vi "from string.vi"(8 "error in":errorcluster, 9 "data":string, 10 "version":string, 11 "Fgen configuration":refnum<class "Fgen configuration.lvclass">) -> (0 "error out":errorcluster, 3 "Fgen configuration out":refnum<class "Fgen configuration.lvclass">)   [LabVIEW 2025, in "Fgen.lvlib" / "Fgen configuration.lvclass"]
doc: "Provides an interface for loading a module configuration from a file or other serialized data source. It is recommended that all children of this class store data in two sets--data required for its own initialization, and any data required for parent initialization--and that each implementation uses the <b>Call Parent Method</b> primitive to de-serialize parent information.Copyright 2017 National Instruments Corporation\n\nLicensed under the Apache License, Version 2.0 (the \"License\"); you may not use this file except in compliance with the License. You may obtain a copy of the License at http://www.apache.org/licenses/LICENSE-2.0\nUnless required by applicable law or agreed to in writing, software distributed under the License is distributed on an \"AS IS\" BASIS, WITHOUT WARRANTIES OR CONDITIONS OF ANY KIND, either express or implied. See the License for the specific language governing permissions and limitations under the License."
uses:
  Fgen configuration.lvclass
  Fgen Setting.ctl
  Fgen configuration.lvclass/Fgen configuration.ctl
  Users/Public/Documents/Sandia National Labs/TSS Plugin/Abstract Engine.lvlibp/Plugin/Abstract/Instrument configuration/Instrument configuration.lvclass
  Users/Public/Documents/Sandia National Labs/TSS Plugin/CEF.lvlibp/serializable configuration/CEF_serializable configuration.lvclass
  Users/Public/Documents/Sandia National Labs/TSS Plugin/CEF.lvlibp
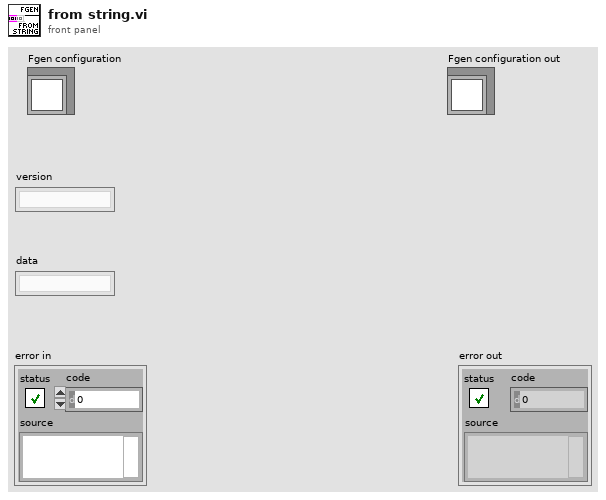
[diagram p1: front panel]
types:
  T1 = typedef "Fgen.lvlib/Fgen configuration.lvclass/Fgen Setting.ctl" = cluster{"Type":string, "Output Mode":string, "Sample Rate":dbl, "Samples":dbl, "Gain":dbl, "Trigger":string, "Impedance":string, "Offset":dbl}
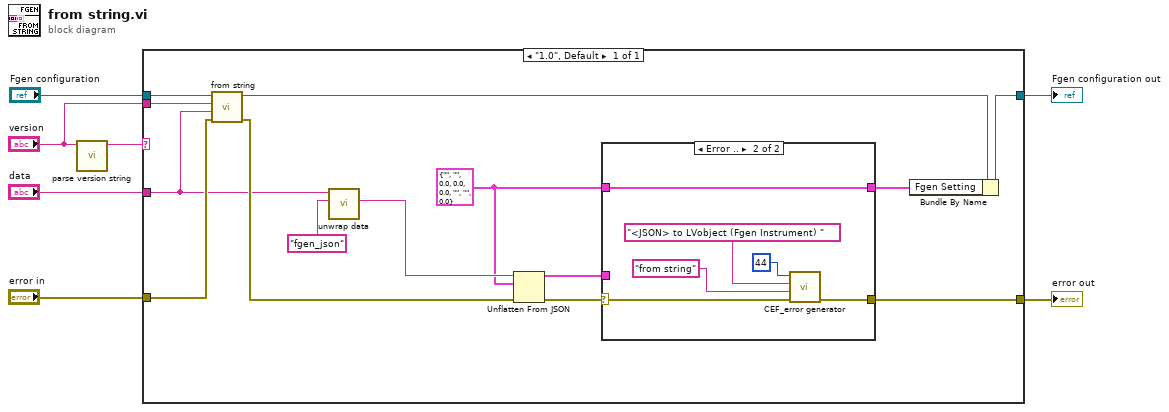
[diagram p0: block diagram]
diagram:
  n1 = call "parse version string.vi"("full version"="version") -> ("major.minor version"=w3:string)  [unwired: 7 in, 3 out]
  n2 = case shown="\"1.0\", Default" w3 {
    tunnel: "Fgen configuration" -> [w21]
    tunnel: [w16] -> w4
    tunnel: "data" -> [w13]
    tunnel: "error in" -> [w18]
    tunnel: "version" -> [w14]
    tunnel: [w8] -> w1
    frame "1.0", Default {
      w12 = T1 {"Type"="", "Output Mode"="", "Sample Rate"=0.0, "Samples"=0.0, "Gain"=0.0, "Trigger"="", "Impedance"="", "Offset"=0.0} ("Setting")
      n3 = call-parent "from string.vi"("error in"=w18, "data"=w13, "version"=w14, "Instrument configuration"=w21) -> ("error out"=w15:errorcluster, "Instrument configuration out"=w20:refnum<class "Fgen configuration.lvclass">)  [unwired: 6 in]
      n4 = call "unwrap data.vi"("identifier"="fgen_json" ("additional identifier"), "data to unwrap"=w13) -> ("unwrapped data"=w17:string)  [unwired: 8 in, 1 out]
      n5 = Unflatten From JSON(JSON string=w17, type and defaults=w12, error in (no error)=w15) -> (value=w10:T1, error out=w11:errorcluster)  [unwired: 4 in]
      n6 = case shown="Error .." w11 {
        selector: w11 -> [w22 w26]
        tunnel: w10 -> [w23 _]
        tunnel: [w23 w25] -> w9
        tunnel: w12 -> [_ w25]
        tunnel: [w22 w24] -> w8
        frame No Error {
        }
        frame Error {
          n7 = call "CEF_error generator.vi"("error in"=w26, "source"="from string" ("message"), "append error message"="<JSON> to LVobject (Fgen Instrument) " ("message"), "error code (0)"=44) -> ("error out"=w24:errorcluster)  [unwired: 5 in]
        }
      }
      n8 = Bundle By Name(cluster=w20, "Fgen Setting"=w9) -> (w16:refnum<class "Fgen configuration.lvclass">)
    }
  }
  "error out" <- w1
  "Fgen configuration out" <- w4
